vi "Set_WebBrowser_Properties.vi"(6 "ContextMenuEnable":bool, 7 "AllowNavigation":bool=TRUE, 8 "error in (no error)":errorcluster, 10 "Visible":bool=TRUE, 11 "WebBrowser_Mgmt in":refnum<class "WebBrowser_Mgmt.lvclass">) -> (0 "error out":errorcluster, 2 "Type":string, 3 "WebBrowser_Mgmt out":refnum<class "WebBrowser_Mgmt.lvclass">)   [LabVIEW 2016, in "WebBrowser_Mgmt.lvclass"]
uses:
  WebBrowser_Mgmt.lvclass
  WebBrowser_Mgmt.lvclass/WebBrowser_Mgmt.ctl
  System.Windows.Forms
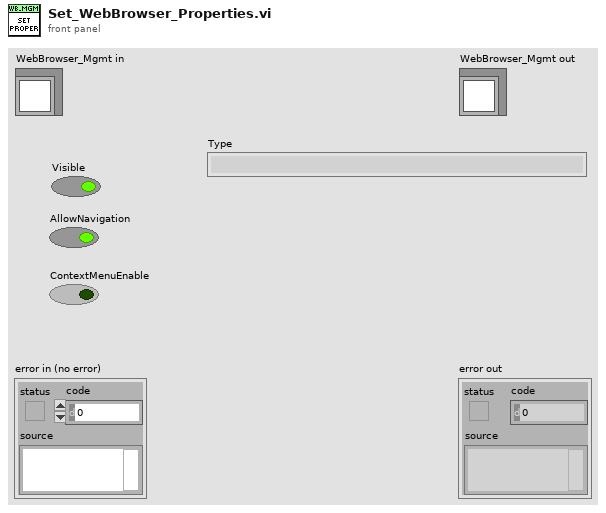
[diagram p1: front panel]
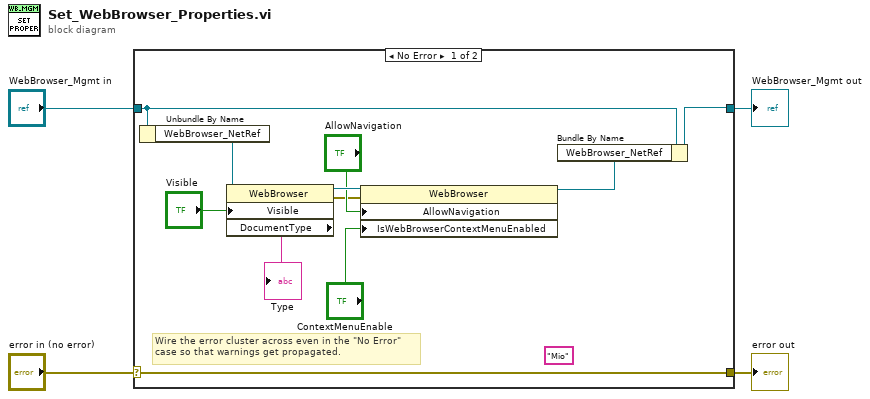
[diagram p0: block diagram]
diagram:
  n1 = case shown="No Error" "error in (no error)" {
    selector: "error in (no error)" -> [w15 w17]
    tunnel: [w15 w17] -> w3
    tunnel: [w6 w16] -> w1
    tunnel: "WebBrowser_Mgmt in" -> [w7 w16]
    frame No Error {
      (unwired) "Mio" ("name")
      # "Wire the error cluster across even in the \"No Error\"\ncase so that warnings get propagated."
      n2 = Unbundle By Name(w7) -> ("WebBrowser_NetRef"=w8:refnum<k24>)
      n3 = property class="WebBrowser"(reference=w8, "Visible"="Visible") -> (reference out=w12:refnum<k24>, error out=w10:errorcluster, "DocumentType"=→"Type":string)  [unwired: 1 in]
      n4 = property class="WebBrowser"(reference=w12, error in=w10, "AllowNavigation"="AllowNavigation", "IsWebBrowserContextMenuEnabled"="ContextMenuEnable") -> (reference out=w5:refnum<k24>)  [unwired: 1 out]
      n5 = Bundle By Name(cluster=w7, "WebBrowser_NetRef"=w5) -> (w6:refnum<class "WebBrowser_Mgmt.lvclass">)
    }
    frame Error {
    }
  }
  "error out" <- w3
  "WebBrowser_Mgmt out" <- w1
